vi "Exercise1.14-Shift Register.vi"() -> ()   [LabVIEW 2013]
panel:
  out "Right Register":i32
  out "Left Register":i32
  out "Left Register":i32
  in  "stop":bool
  out "Right Register":i32
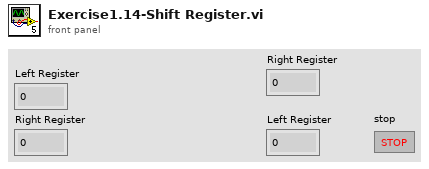
[diagram p1: front panel]
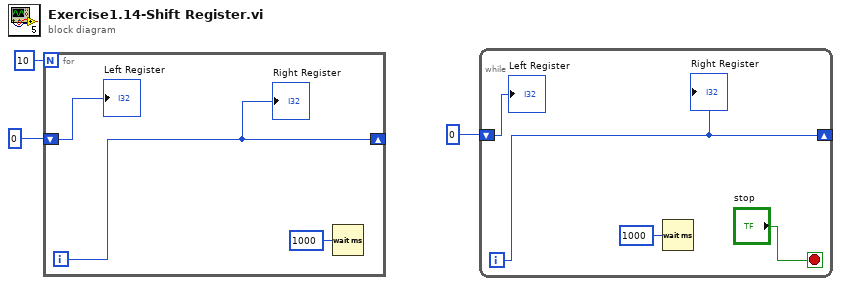
[diagram p0: block diagram]
diagram:
  n1 = for {
    N: 10 -> [_]
    shift-right: [w5] -> _
    shift-left: 0 -> [w6]
    i -> [w5]
    n2 = Wait (ms)(milliseconds to wait=u32 1000) -> ()  [unwired: 1 out]
    "Left Register" <- w6
    "Right Register" <- w5
  }
  n3 = while {
    shift-right: [w10] -> _
    shift-left: 0 -> [w7]
    i -> [w10]
    stop <- "stop" stop-if-true
    n4 = Wait (ms)(milliseconds to wait=u32 1000) -> ()  [unwired: 1 out]
    "Right Register" <- w10
    "Left Register" <- w7
  }
